vi "RH_PPMU_Initialize.vi"(7 "error in":errorcluster, 9 "pin map file":path caption="pin map file path", 10 "PPMU Resource Name":refnum<k15>="Digital1") -> (0 "error out":errorcluster, 3 "PPMU Session Out":refnum<k15>)   [LabVIEW 2023, in "ResourceHandling.lvlib"]
doc: "Initializes PPMU"
uses:
  ResourceHandling.lvlib
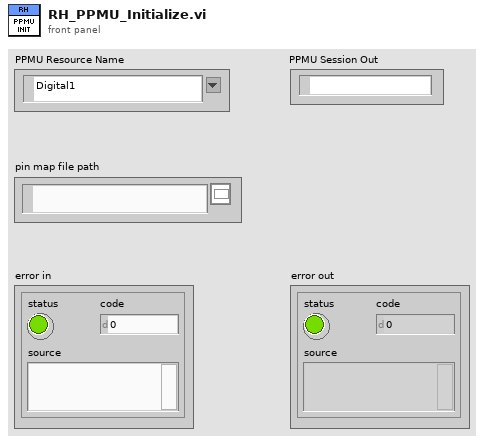
[diagram p1: front panel]
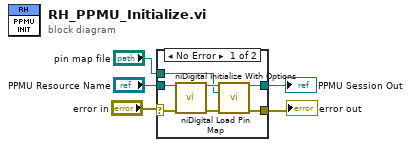
[diagram p0: block diagram]
diagram:
  n1 = case shown="No Error" "error in" {
    selector: "error in" -> [w6 w13]
    tunnel: "PPMU Resource Name" -> [w8 _]
    tunnel: "pin map file" -> [w7 _]
    tunnel: [w9 w13] -> w1
    tunnel: [w10 _] -> w3
    frame No Error {
      n2 = call <instrlib>:"niDigital Initialize With Options.vi"("resource name"=w8, "error in"=w6) -> ("instrument handle"=w12:refnum<k15>, "error out"=w11:errorcluster)  [unwired: 12 in]
      n3 = call <instrlib>:"niDigital Load Pin Map.vi"("instrument handle"=w12, "pin map file"=w7, "error in"=w11) -> ("instrument handle out"=w10:refnum<k15>, "error out"=w9:errorcluster)  [unwired: 11 in]
    }
    frame Error {
    }
  }
  "PPMU Session Out" <- w3
  "error out" <- w1
